vi "loading.vi"(11 "VISA resource name":refnum<visa-resource-name>) -> ()   [LabVIEW 2020]
panel:
  out "LoadCell":dbl
  # "kgf"
  # "LOADGIND..."
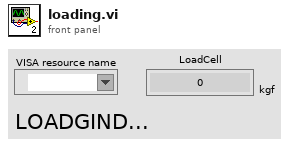
[diagram p1: front panel]
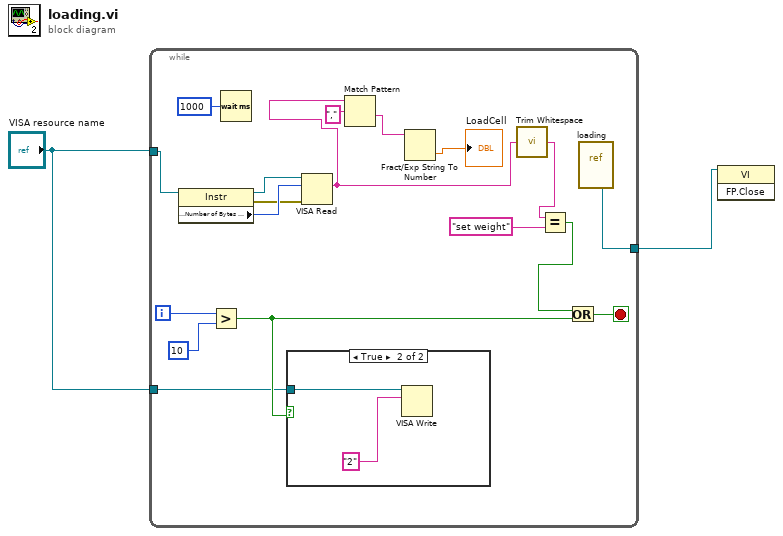
[diagram p0: block diagram]
diagram:
  n1 = while {
    tunnel: "VISA resource name" -> [w17]
    tunnel: [w5] -> w2
    tunnel: "VISA resource name" -> [w3]
    i -> [w14]
    stop <- w11 stop-if-true
    n2 = property class="Instr"(reference=w17) -> (reference out=w19:refnum<visa-resource-name>, error out=w18:errorcluster, "Serial Settings:Number of Bytes at Serial Port"=w20:u32)  [unwired: 1 in]
    n3 = Greater?(x=w14, y=10) -> (0:w4:bool)
    n4 = Wait (ms)(milliseconds to wait=u32 1000) -> ()  [unwired: 1 out]
    n5 = case shown="True" w4 {
      tunnel: w3 -> [_ w21]
      frame False {
      }
      frame True {
        n6 = VISA Write(VISA resource name=w21, write buffer="2") -> ()  [unwired: 1 in, 3 out]
      }
    }
    n7 = VISA Read(VISA resource name=w19, byte count=w20, error in (no error)=w18) -> (read buffer=w6:string)  [unwired: 3 out]
    n8 = Match Pattern(string=w6, regular expression="," ("정규식")) -> (after substring=w8:string)  [unwired: 1 in, 3 out]
    n9 = Fract/Exp String To Number(string=w8) -> (number=→"LoadCell":dbl)  [unwired: 3 in, 1 out]
    n10 = call <vilib>:"Trim Whitespace.vi"("string"=w6) -> ("trimmed string"=w16:string)  [unwired: 1 in]
    n11 = Equal?(x=w16, y="set weight") -> (x = y?=w12:bool)
    n12 = Or(x=w12, y=w4) -> (x .or. y?=w11:bool)
    n13 = vi-ref "loading.vi"() -> (w5:refnum<vi>)
  }
  n14 = invoke class="VI" method="FP.Close"(reference=w2) -> ()  [unwired: 2 in, 3 out]
